vi "IKPI_Parse_Logging.vi"() -> ()   [LabVIEW 2019]
uses:
  <vilib>/Instr/_visa.llb/VISA Configure Serial Port (Instr).vi
  <vilib>/Utility/file.llb/Write Delimited Spreadsheet (string).vi
panel:
  in  "Checkbox":bool
  out "String":string
  in  "file path (dialog if empty)":path
  in  "Input User":string
  out "Waveform Chart":cluster{i32, i32}(graph)
  in  "stop":bool
  out "error out":errorcluster
  in  "Select Port":refnum<visa-resource-name>
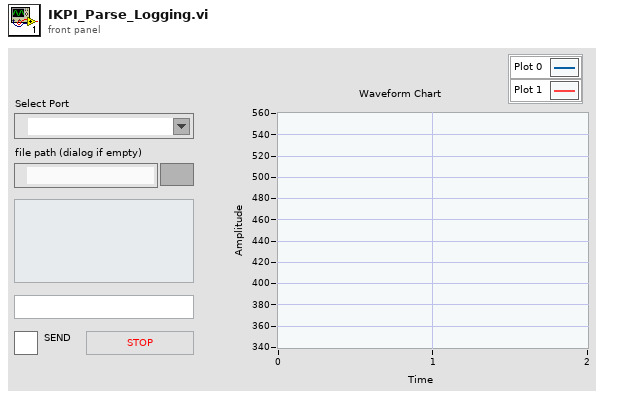
[diagram p1: front panel]
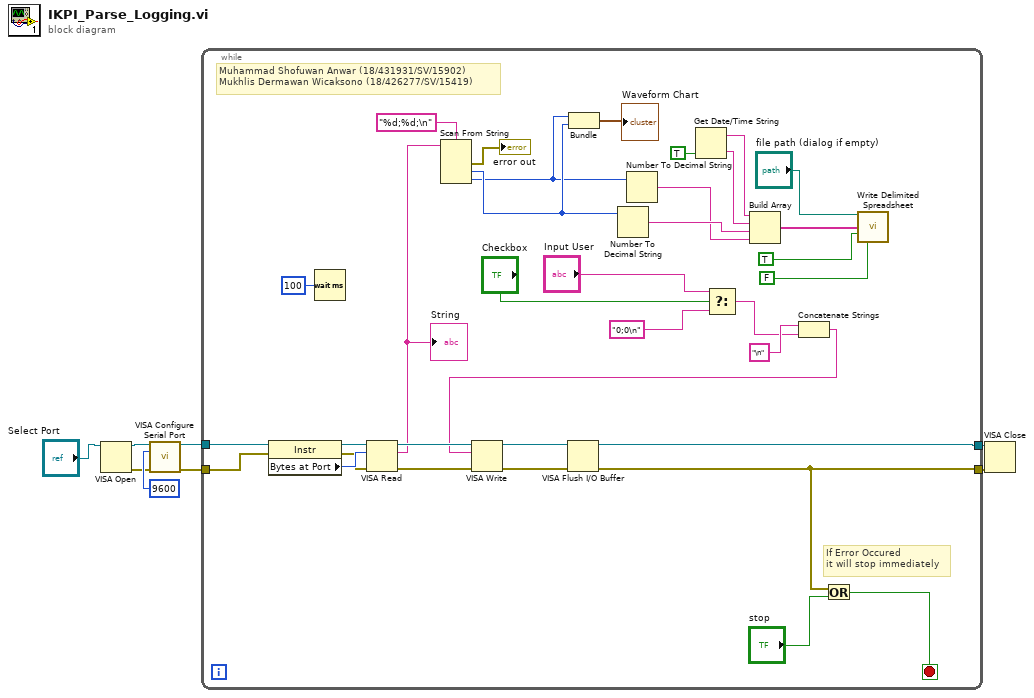
[diagram p0: block diagram]
diagram:
  n1 = VISA Open(VISA resource name="Select Port") -> (VISA resource name=w4:refnum<visa-resource-name>, error out=w5:errorcluster)  [unwired: 4 in]
  n2 = call-poly "VISA Configure Serial Port"("VISA resource name"=w4, "baud rate (9600)"=u32 9600, "error in (no error)"=w5) -> ("VISA resource name out"=w7:refnum<visa-resource-name>, "error out"=w6:errorcluster)  [unwired: 11 in]
  n3 = while {
    tunnel: w7 -> [w43]
    tunnel: w6 -> [w42]
    tunnel: [w31] -> w2
    tunnel: [w30] -> w1
    stop <- w36 stop-if-true
    # "Muhammad Shofuwan Anwar (18/431931/SV/15902)\nMukhlis Dermawan Wicaksono (18/426277/SV/15419)"
    # "If Error Occured\nit will stop immediately"
    n4 = property class="Instr"(reference=w43, error in=w42) -> (reference out=w40:refnum<visa-resource-name>, error out=w39:errorcluster, "Bytes at Port"=w41:u32)
    n5 = Wait (ms)(milliseconds to wait=u32 100) -> ()  [unwired: 1 out]
    n6 = VISA Read(VISA resource name=w40, byte count=w41, error in (no error)=w39) -> (VISA resource name out=w38:refnum<visa-resource-name>, read buffer=w20:string, error out=w37:errorcluster)  [unwired: 1 out]
    "String" <- w20
    n7 = Scan From String(format string="%d;%d;\n", input string=w20) -> (error out=→"error out":errorcluster, output 1=w16:i32, output 2=w15:i32)  [unwired: 4 in, 2 out]
    n8 = Bundle(w15, w16) -> (→"Waveform Chart":cluster{i32, i32})  [unwired: 1 in]
    n9 = Number To Decimal String(number=w16) -> (decimal integer string=w10:string)  [unwired: 1 in]
    n10 = Number To Decimal String(number=w15) -> (decimal integer string=w9:string)  [unwired: 1 in]
    n11 = Get Date/Time String(want seconds? (F)=TRUE) -> (date string=w24:string, time string=w25:string)  [unwired: 2 in]
    n12 = Select(t="Input User", s="Checkbox", f="0;0\n") -> (s? t:f=w11:string)
    n13 = Build Array(w24, w25, w10, w9) -> (w27:string[])
    n14 = Concatenate Strings("\n" ("string"), w11) -> (w13:string)
    n15 = VISA Write(VISA resource name=w38, write buffer=w13, error in (no error)=w37) -> (VISA resource name out=w33:refnum<visa-resource-name>, error out=w32:errorcluster)  [unwired: 1 out]
    n16 = VISA Flush I/O Buffer(VISA resource name=w33, error in (no error)=w32) -> (VISA resource name out=w31:refnum<visa-resource-name>, error out=w30:errorcluster)  [unwired: 1 in]
    n17 = Or(x=w30, y="stop") -> (x .or. y?=w36:bool)
    n18 = call-poly <vilib>:"Write Delimited Spreadsheet.vi"("file path (dialog if empty)"="file path (dialog if empty)", "1D data"=w27, "append to file? (new file:F)"=TRUE, "transpose? (no:F)"=FALSE) -> ()  [unwired: 10 in, 2 out]
  }
  n19 = VISA Close(VISA resource name=w2, error in (no error)=w1) -> ()  [unwired: 1 out]
